vi "Get Stream Position.vi"(8 "error in (no error)":errorcluster, 11 "Stream in":refnum<class "Stream.lvclass">) -> (0 "error out":errorcluster, 2 "Position":i64, 3 "Stream out":refnum<class "Stream.lvclass">)   [LabVIEW 2020, in "Stream.lvlib" / "Stream.lvclass"]
uses:
  Stream.lvclass
  Stream.lvlib
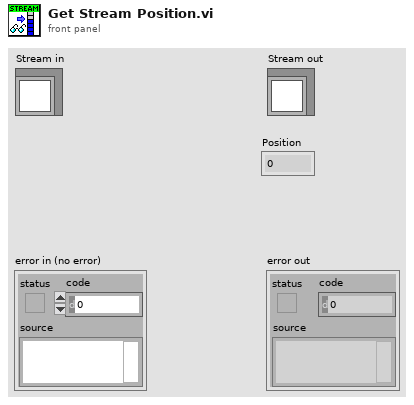
[diagram p1: front panel]
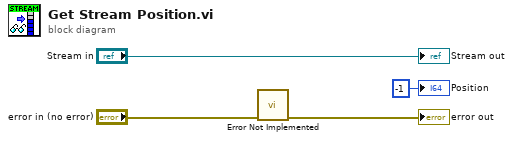
[diagram p0: block diagram]
diagram:
  n1 = call "Error Not Implemented.vi"("error in (no error)"="error in (no error)") -> ("error out"=→"error out":errorcluster)  [unwired: 10 in]
  "Stream out" <- "Stream in"
  "Position" <- i64 -1 ("Position")
